vi "hdfTest.vi"() -> ()   [LabVIEW 2017]
uses:
  <vilib>/UPVI/lvhdf5/dataset.llb/LVH5D Operation.ctl
  <vilib>/Utility/miscctls.llb/LVRectTypeDef.ctl
  <vilib>/UPVI/lvhdf5/attribute.llb/LVH5A Operation.ctl
  <vilib>/UPVI/lvhdf5/group.llb/H5G_obj_t.ctl
  <vilib>/UPVI/lvhdf5/file.llb/LVH5F Operation.ctl
  <vilib>/UPVI/lvhdf5/identifier.llb/Not an HDF5 Refnum Constant.vi
  <vilib>/UPVI/lvhdf5/common.llb/To HDF5 Ref.vi
  <vilib>/UPVI/lvhdf5/file.llb/OpenCreateReplace HDF5 File.vi
  <vilib>/UPVI/lvhdf5/utility.llb/Select HDF5 Dialog.vi
  <vilib>/UPVI/lvhdf5/utility.llb/Select HDF5 Dialog (File and Object).vi
  <vilib>/UPVI/lvhdf5/dataset.llb/Simple H5Dwrite (Variant).vi
  <vilib>/UPVI/lvhdf5/attribute.llb/Write Multiple Attributes.vi
  <vilib>/UPVI/lvhdf5/dataset.llb/H5Dclose.vi
  <vilib>/UPVI/lvhdf5/dataset.llb/Write Dataset with Attributes.xnode
  <vilib>/UPVI/lvhdf5/library.llb/HDF5 Ref.ctl
  <vilib>/Analysis/NI_AALBase.lvlib
  <vilib>/Utility/error.llb/Error Cluster From Error Code.vi
  <vilib>/UPVI/lvhdf5/dataset.llb/OpenCreateReplace Dataset by Element Type.vi
  <vilib>/UPVI/lvhdf5/dataspace.llb/H5Sselect_hyperslab.vi
  <vilib>/UPVI/lvhdf5/dataset.llb/H5Dwrite (Variant).vi
  <vilib>/UPVI/lvhdf5/dataset.llb/H5Dget_space.vi
  <vilib>/UPVI/lvhdf5/attribute.llb/private/LVH5AwriteWDTAttrs.vi
  <vilib>/UPVI/lvhdf5/dataspace.llb/H5Sclose.vi
  <vilib>/UPVI/lvhdf5/utility.llb/Select HDF5 Dialog (Object Only).vi
  <vilib>/Utility/VariantDataType/GetClusterInfo.vi
  <vilib>/Utility/VariantDataType/VariantType.lvlib
  <vilib>/Utility/VariantDataType/GetTypeInfo.vi
  <vilib>/UPVI/lvhdf5/attribute.llb/Cluster to Attribute Array.xnode
panel:
  out "Array":dbl[][](array[numeric])
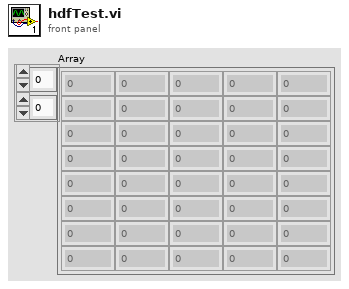
[diagram p1: front panel]
types:
  T1 = typedef "LVH5D Operation.ctl" = enum16{"open", "replace", "create", "open or create", "create or replace", "create or replace with confirmation"}
  T2 = typedef "HDF5 Ref.ctl" = refnum<k1>
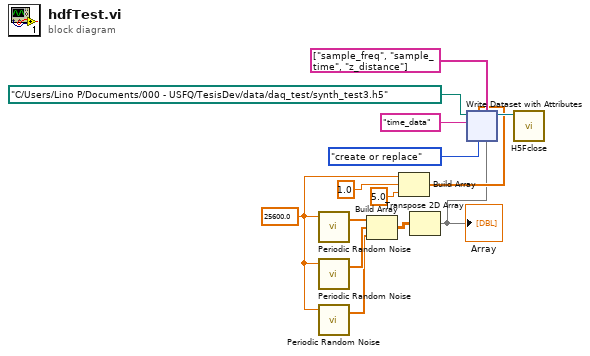
[diagram p0: block diagram]
diagram:
  w2 = 25600.0 ("rate")
  n1 = call <vilib>:"Periodic Random Noise.vi"("samples"=w2) -> ("periodic random noise"=w8:dbl[])  [unwired: 2 in, 1 out]
  n2 = call <vilib>:"Periodic Random Noise.vi"("samples"=w2) -> ("periodic random noise"=w7:dbl[])  [unwired: 2 in, 1 out]
  n3 = call <vilib>:"Periodic Random Noise.vi"("samples"=w2) -> ("periodic random noise"=w1:dbl[])  [unwired: 2 in, 1 out]
  n4 = Build Array(w8, w7, w1) -> (w6:dbl[][])
  n5 = Build Array(w2, 1.0 ("element"), 5.0 ("element")) -> (w9:dbl[])
  n6 = Transpose 2D Array(2D array=w6) -> (transposed array=w5:dbl[][])
  "Array" <- w5
  n7 = xnode "Write Dataset with Attributes"("Dataset Path"="time_data", "operation (open or create)"=LVH5D_Operation."create or replace", "HDF5 Path or Ref"=path "C:/Users/Lino P/Documents/000 - USFQ/TesisDev/data/daq_test/synth_test3.h5" ("path"), "Attribute Name(s)"=string[] ["sample_freq", "sample_time", "z_distance"], "Attribute Value(s)"=w9, "Data"=w5) -> ("HDF5 Ref out"=w11:T2)  [unwired: 2 in, 2 out]
  n8 = call <vilib>:"H5Fclose.vi"("HDF5 Ref"=w11) -> ()  [unwired: 8 in, 1 out]
